vi "Wait For Acquisition Complete.vi"(8 "error in (no error)":errorcluster, 10 "Timeout (10000 ms)":u32=10000, 11 "VISA resource name":refnum<visa-resource-name>) -> (0 "error out":errorcluster, 2 "Complete":bool, 3 "VISA resource name out":refnum<visa-resource-name>)   [LabVIEW 2018, in "LeCroy Wave Series.lvlib"]
doc: "This detect whether previous operation finished in specified time or no."
uses:
  LeCroy Wave Series.lvlib
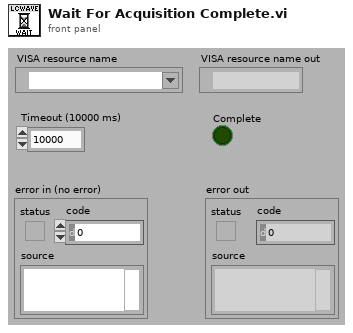
[diagram p1: front panel]
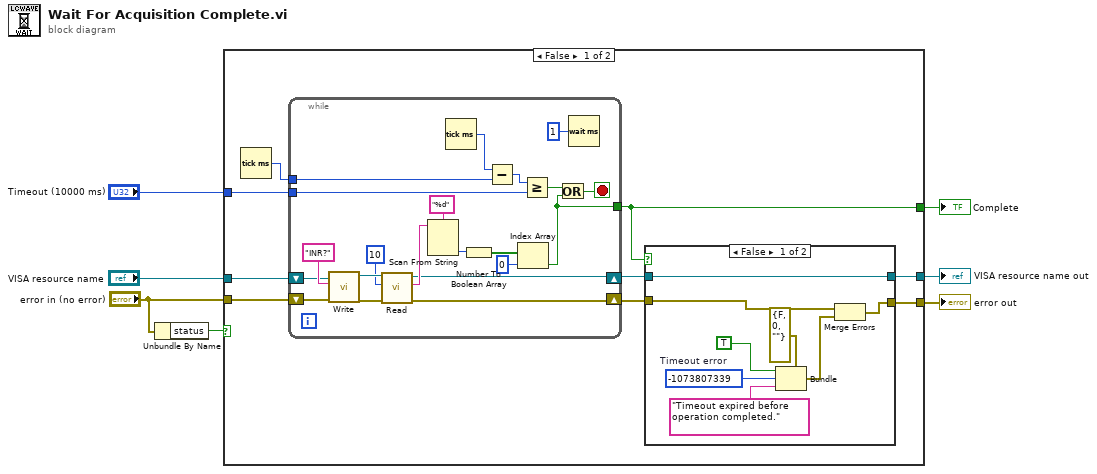
[diagram p0: block diagram]
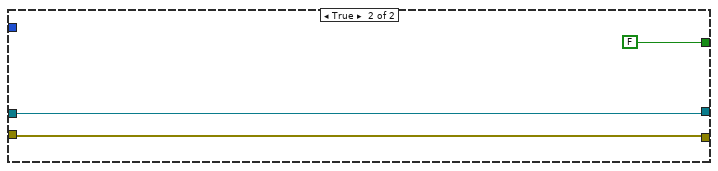
[diagram p3: hidden frame]
diagram:
  n1 = Unbundle By Name("error in (no error)") -> ("status"=w2:bool)
  n2 = case shown="False" w2 {
    tunnel: "VISA resource name" -> [w16 w50]
    tunnel: "Timeout (10000 ms)" -> [w14 _]
    tunnel: [w11 w50] -> w5
    tunnel: [w10 w49] -> w4
    tunnel: "error in (no error)" -> [w9 w49]
    tunnel: [w8 FALSE] -> w1
    frame False {
      n3 = Tick Count (ms)() -> (millisecond timer value=w15:u32)
      n4 = while {
        tunnel: w15 -> [w35]
        tunnel: w14 -> [w33]
        tunnel: [w30] -> w8
        shift-right: [w28] -> w13
        shift-left: w16 -> [w38]
        shift-right: [w27] -> w12
        shift-left: w9 -> [w37]
        stop <- w32 stop-if-true
        n5 = call "Write.vi"("error in (no error)"=w37, "Write Buffer"="INR?" ("write buffer"), "VISA resource name"=w38) -> ("error out"=w46:errorcluster, "VISA resource name out"=w47:refnum<visa-resource-name>)  [unwired: 6 in, 1 out]
        n6 = call "Read.vi"("error in (no error)"=w46, "Byte Count"=u32 10 ("byte count"), "VISA resource name"=w47) -> ("error out"=w27:errorcluster, "Read Buffer"=w44:string, "VISA resource name out"=w28:refnum<visa-resource-name>)  [unwired: 5 in, 1 out]
        n7 = Scan From String(format string="%d", input string=w44) -> (output 1=w41:i32)  [unwired: 3 in, 3 out]
        n8 = Tick Count (ms)() -> (millisecond timer value=w36:u32)
        n9 = Number To Boolean Array(number=w41) -> (Boolean array=w40:bool[])
        n10 = Subtract(x=w36, y=w35) -> (x-y=w34:u32)
        n11 = Index Array(array=w40, index=0) -> (element=w30:bool)
        n12 = Greater Or Equal?(x=w34, y=w33) -> (x >= y?=w31:bool)
        n13 = Or(x=w31, y=w30) -> (x .or. y?=w32:bool)
        n14 = Wait (ms)(milliseconds to wait=u32 1) -> ()  [unwired: 1 out]
      }
      n15 = case shown="False" w8 {
        tunnel: w13 -> [w20 w26]
        tunnel: w12 -> [w18 w25]
        tunnel: [w20 w26] -> w11
        tunnel: [w19 w25] -> w10
        frame False {
          w23 = -1073807339  # Timeout error
          n16 = Bundle(cluster=errorcluster {"status"=FALSE, "code"=0, "source"=""} ("error out"), "status"=TRUE, "code"=w23, "source"="Timeout expired before operation completed." ("Source")) -> (w17:errorcluster)
          n17 = Merge Errors(w18, w17) -> (w19:errorcluster)
        }
        frame True {
        }
      }
    }
    frame True {
    }
  }
  "VISA resource name out" <- w5
  "error out" <- w4
  "Complete" <- w1
